vi "Read_Local_ini_Key.vi"(8 "Error In":errorcluster, 11 "Local ini path":path) -> (0 "Error Out":errorcluster, 2 "cluster":T1)   [LabVIEW 2017]
doc: "This subVI fetches all the parameters from the local ini file and parameters are relevant to test case.\n\n<B>Path:</B>\n\\\\UltraSonic_Test_Scripts\\\\BF_INT_TESTSUITE_AUTO\\\\testcasename\\\\testcasename.ini\n\n<B>For Ex:</B>\nuserid=ADMIN\npassword=123456Aa#\nrequests_url_command=http://192.168.2.101/login\nPOST_Data_command={\"Sid\":12345}\nIterations=1\nDelayBetweenIterations=1000 in ms\nTimeout=15000 in ms\nTimestamp=14052019_0341 \nTestSuite=BF_INT_WEBSERVICES_AUTO"
uses:
  <vilib>/Utility/config.llb/Read Key (String).vi
  <vilib>/Utility/config.llb/NI_LVConfig.lvlib
panel:
  out "file created?":bool
  out "error out":errorcluster
  out "section names":string[](array[string])
  out "Keys in ini":string[](array[string])
  # "READ FROM LOCAL INI FILE"
  # "ERROR"
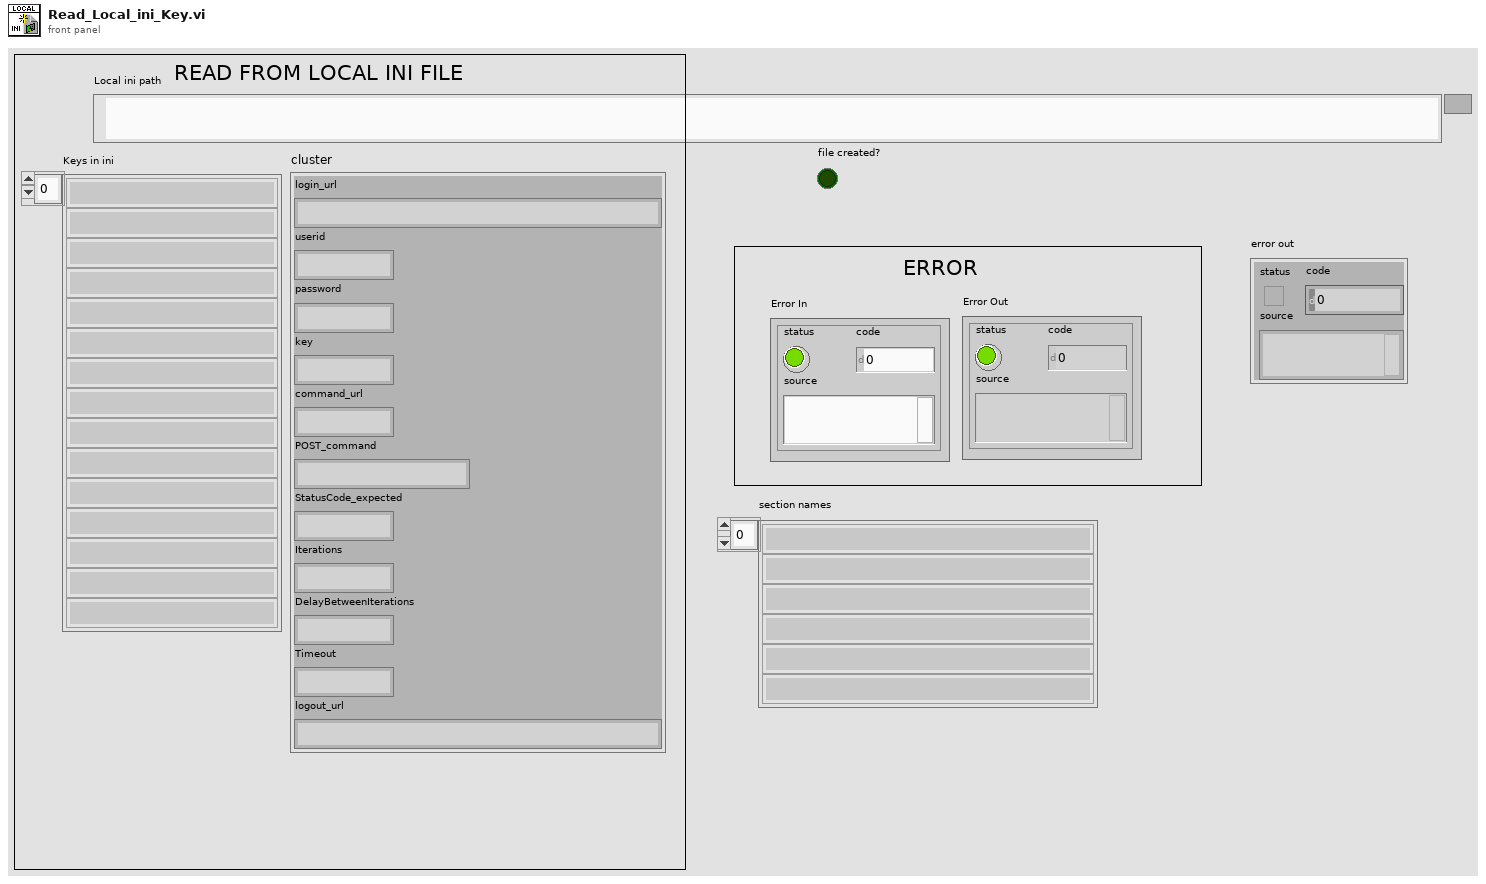
[diagram p1: front panel]
types:
  T1 = cluster{"login_url":string, "userid":string, "password":string, "key":string, "command_url":string, "POST_command":string, "StatusCode_expected":string, "Iterations":string, "DelayBetweenIterations":string, "Timeout":string, "logout_url":string}
  T2 = typedef "NI_LVConfig.lvlib/Config Data RefNum.ctl" = refnum<k1>
  T3 = cluster{"[0]":string, "[1]":string, "[2]":string, "[3]":string, "[4]":string, "[5]":string, "[6]":string, "[7]":string, "[8]":string, "[9]":string, "[10]":string}
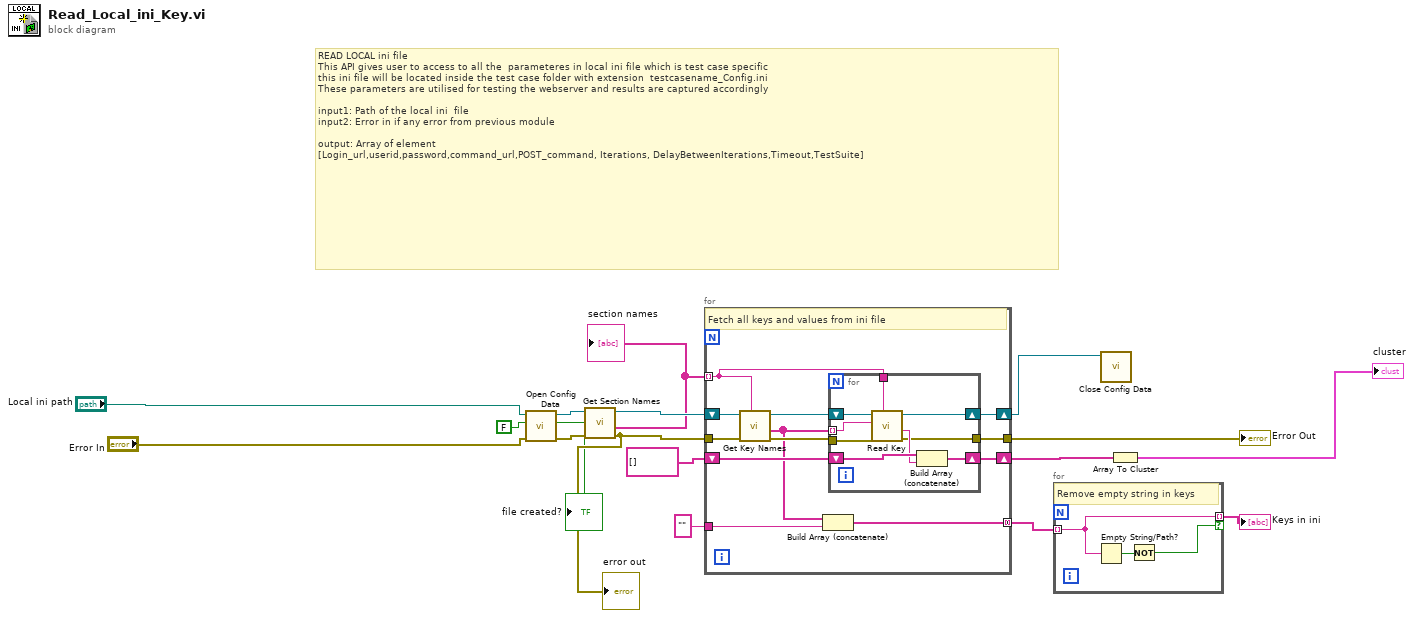
[diagram p0: block diagram]
diagram:
  # "READ LOCAL ini file\nThis API gives user to access to all the  parameteres in local ini file which is test case specific\nthis ini file will be located inside the test case folder with extension  testcasename_Config.ini\nThese parameters are utilised for testing the webserver and results are captured accordingly\n\ninput1: Path of the local ini  file\ninput2: Error in if any error from previous module\n\noutput: Array of element\n[Login_url,userid,password,command_url,POST_command, Iterations, DelayBetweenIterations,Timeout,TestSuite]"
  n1 = call <vilib>:"Open Config Data.vi"("error in (no error)"="Error In", "create file if necessary (T)"=FALSE ("create file if necessary? (T)"), "configuration file path"="Local ini path") -> ("error out"=w12:errorcluster, "file created?"=→"file created?":bool, "refnum"=w14:T2)  [unwired: 6 in]
  n2 = call <vilib>:"Get Section Names.vi"("error in (no error)"=w12, "refnum"=w14) -> ("error out"=w4:errorcluster, "section names"=w11:string[], "refnum out"=w13:T2)  [unwired: 7 in]
  "section names" <- w11
  "error out" <- w4
  n3 = for {
    tunnel: w4 -> [w26]
    tunnel: w11 -> [w25] mode=indexing
    shift-right: [w24] -> w6
    shift-left: string[] [] -> [w23]
    tunnel: "" -> [w21]
    tunnel: [w20] -> w8 mode=concatenating
    tunnel: [w19] -> w5
    shift-right: [w18] -> w2
    shift-left: w13 -> [w27]
    # "Fetch all keys and values from ini file"
    n4 = call <vilib>:"Get Key Names.vi"("section"=w25, "error in (no error)"=w26, "refnum"=w27) -> ("error out"=w28:errorcluster, "key names"=w22:string[], "refnum out"=w29:T2)  [unwired: 5 in, 1 out]
    n5 = Build Array (concatenate)(w22, w21) -> (w20:string[])
    n6 = for {
      tunnel: w22 -> [w34] mode=indexing
      tunnel: w28 -> [w37]
      shift-right: [w36] -> w24
      shift-left: w23 -> [w33]
      tunnel: w25 -> [w35]
      tunnel: [w31] -> w19
      shift-right: [w30] -> w18
      shift-left: w29 -> [w38]
      n7 = call-poly <vilib>:"Read Key.vi"("section"=w35, "error in (no error)"=w37, "key"=w34, "refnum"=w38) -> ("error out"=w31:errorcluster, "value"=w32:string, "refnum out"=w30:T2)  [unwired: 2 in, 3 out]
      n8 = Build Array (concatenate)(w33, w32) -> (w36:string[])
    }
  }
  "Error Out" <- w5
  n9 = for {
    tunnel: w8 -> [w40] mode=indexing
    tunnel: [w40] -> w7 mode=indexing if=w39
    # "Remove empty string in keys"
    n10 = Empty String/Path?(string/path=w40) -> (empty?=w41:bool)
    n11 = Not(x=w41) -> (.not. x?=w39:bool)
  }
  "Keys in ini" <- w7
  n12 = call <vilib>:"Close Config Data.vi"("refnum"=w2) -> ()  [unwired: 9 in, 2 out]
  n13 = Array To Cluster(array=w6) -> (cluster=→"cluster":T3)
